vi "Eurotherm test MAX FPGA B.vi"() -> ()   [LabVIEW 2011]
uses:
  <vilib>/rvi/eio/common/nirviEmuTemplateMethod_errors.vi
  <vilib>/eio/EIOMethodNode/EIOMethodNode.xnode
panel:
  in  "Command":i16
  in  "Ramp rate SP&CRC":u8[](array[numeric])=[66, 0, 0, 0, 132, 246]
  in  "SP&CRC":u8[](array[numeric])=[65, 32, 0, 0, 133, 120]
  # "0 - Set point\n1 - Rap rate"
  # "10deg\n65\n32\n0\n0\n133\n120"
  # "50deg\n66\n200\n0\n0\n5\n8"
  # "10deg\n65\n32\n0\n0\n3\n133"
  # "50deg\n66\n72\n0\n0\n130\n29"
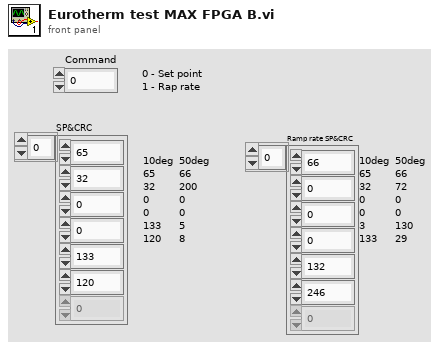
[diagram p1: front panel]
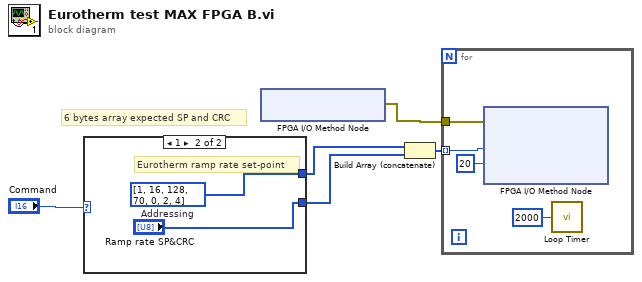
[diagram p0: block diagram]
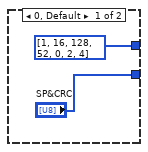
[diagram p2: hidden frame]
diagram:
  # "6 bytes array expected SP and CRC"
  n1 = case shown="1" "Command" {
    tunnel: [u8[] [1, 16, 128, 52, 0, 2, 4] ("Addressing") w9] -> w5
    tunnel: ["SP&CRC" "Ramp rate SP&CRC"] -> w4
    frame 0, Default {
    }
    frame 1 {
      w9 = u8[] [1, 16, 128, 70, 0, 2, 4]  # Addressing
      # "Eurotherm ramp rate set-point"
    }
  }
  n2 = xnode "FPGA I/O Method Node"() -> ("error out"=w3:errorcluster)  [unwired: 2 in, 1 out]
  n3 = Build Array (concatenate)(w5, w4) -> (w2:u8[])
  n4 = for {
    tunnel: w3 -> [w13]
    tunnel: w2 -> [w12] mode=indexing
    n5 = xnode "FPGA I/O Method Node"("error in"=w13, "Data"=w12, "Timeout (ms)"=20) -> ()  [unwired: 1 in, 3 out]
    n6 = call "Loop Timer"("Count(uSec)"=u32 2000) -> ()  [unwired: 1 out]
  }
